vi "CalcNewPos.vi"(3 "New UTM Location":T1 {"North" format="%#_10f"; "East" format="%#_8f"}, 8 "Current UTM Location":T1 {"North" format="%#_10f"; "East" format="%#_8f"}, 9 "dt":dbl, 10 "Robot Velocity":dbl, 11 "Robot Heading":dbl) -> ()   [LabVIEW 2012]
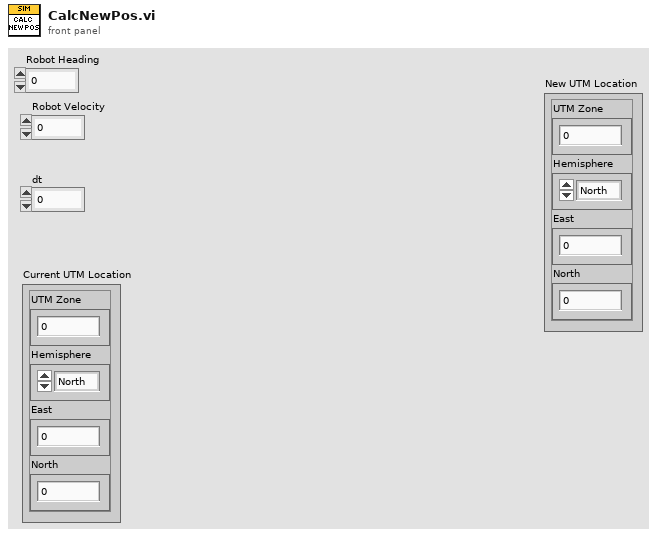
[diagram p1: front panel]
types:
  T1 = cluster{"UTM Zone":dbl, "Hemisphere":enum16{"North", "South"}, "East":dbl, "North":dbl}
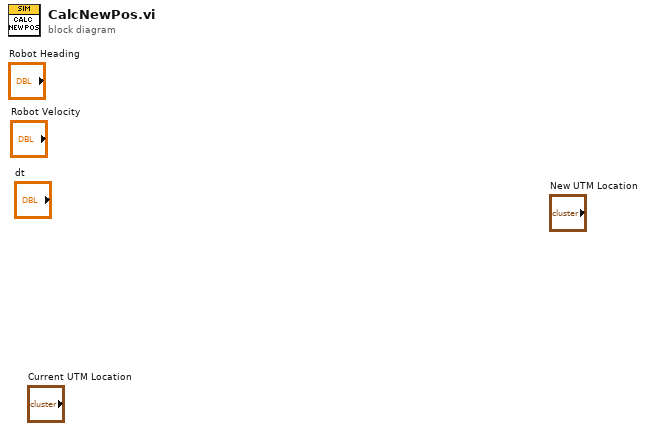
[diagram p0: block diagram]
diagram:
